vi "Move Up Channel in Wfm Grp.vi"(7 "Channels Ctrl Ref":refnum<vi>, 8 "error in (no error)":errorcluster, 11 "To Save Wfm Arrays":waveform(dbl)[](array[waveform])) -> (0 "error out":errorcluster, 3 "Wfm Grp Data":T1)   [LabVIEW 2025, in "TDMS Waveform Creator UI.lvlib"]
uses:
  TDMS Waveform Creator UI.lvlib
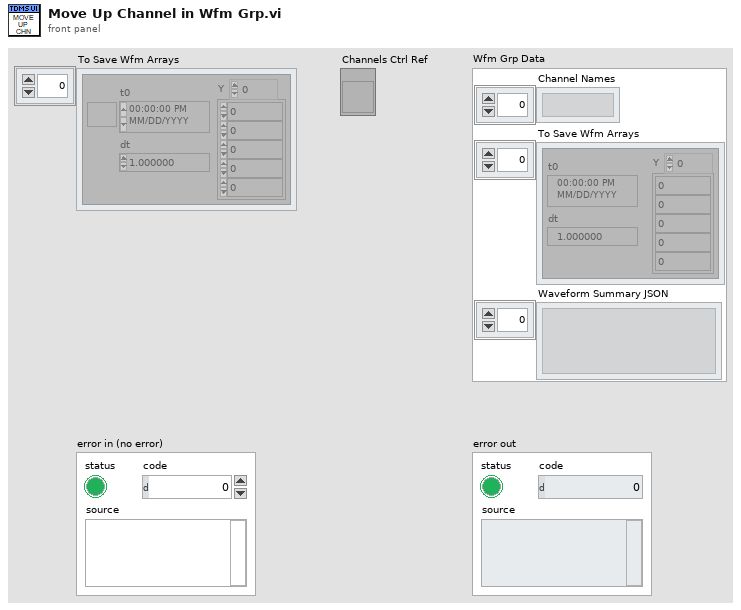
[diagram p1: front panel]
types:
  T1 = cluster{"Channel Names":string[], "To Save Wfm Arrays":waveform(dbl)[], "Waveform Summary JSON":string[]}
  T2 = cluster{"Item Names":string[], waveform(dbl)[], string[]}
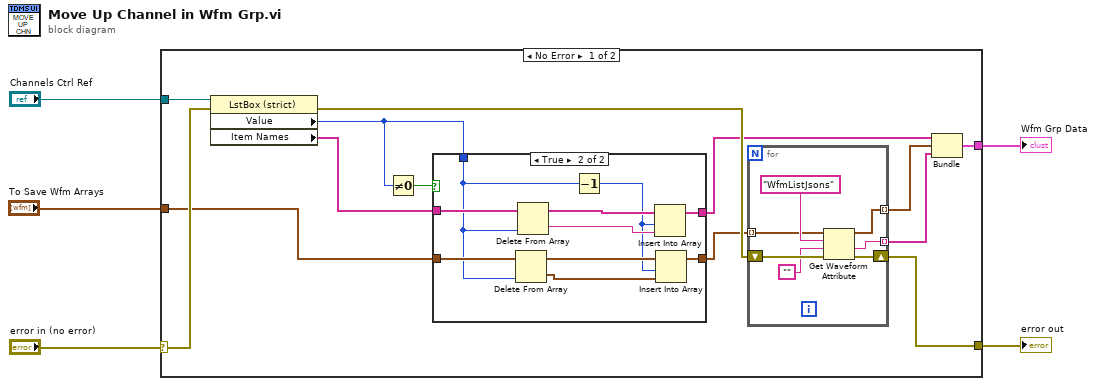
[diagram p0: block diagram]
diagram:
  n1 = case shown="No Error" "error in (no error)" {
    selector: "error in (no error)" -> [w17 w38]
    tunnel: "Channels Ctrl Ref" -> [w18 _]
    tunnel: "To Save Wfm Arrays" -> [w8 _]
    tunnel: [w15 w38] -> w2
    tunnel: [w12 _] -> w1
    frame No Error {
      n2 = property class="LstBox (strict)"(reference=w18, error in=w17) -> (error out=w16:errorcluster, "Value"=w10:i32, "Item Names"=w11:string[])  [unwired: 1 out]
      n3 = Not Equal To 0?(x=w10) -> (x != 0?=w9:bool)
      n4 = case shown="True" w9 {
        tunnel: w11 -> [w27 w37]
        tunnel: w8 -> [w26 w34]
        tunnel: w10 -> [_ w33]
        tunnel: [w27 w32] -> w6
        tunnel: [w26 w30] -> w7
        frame False {
        }
        frame True {
          n5 = Delete From Array(array=w34, index=w33) -> (deleted portion=w29:waveform(dbl), array with subset deleted=w36:waveform(dbl)[])  [unwired: 1 in]
          n6 = Delete From Array(array=w37, index=w33) -> (deleted portion=w31:string, array with subset deleted=w35:string[])  [unwired: 1 in]
          n7 = Decrement(x=w33) -> (x-1=w28:i32)
          n8 = Insert Into Array(array=w35, index=w28, new element=w31) -> (w32:string[])
          n9 = Insert Into Array(array=w36, index=w28, new element=w29) -> (w30:waveform(dbl)[])
        }
      }
      n10 = for {
        shift-right: [w24] -> w15
        shift-left: w16 -> [w25]
        tunnel: [w23] -> w14 mode=indexing
        tunnel: [w20] -> w13 mode=indexing
        tunnel: w7 -> [w19] mode=indexing
        n11 = Get Waveform Attribute(4:w25, 5:"", 6:"WfmListJsons" ("name"), 7:w19) -> (0:w24:errorcluster, 1:w20:string, 3:w23:waveform(dbl))  [unwired: 1 out]
      }
      n12 = Bundle("Item Names"=w6, w14, w13) -> (w12:T2)  [unwired: 1 in]
    }
    frame Error {
    }
  }
  "error out" <- w2
  "Wfm Grp Data" <- w1
